vi "Imagen_BN.vi"() -> ()   [LabVIEW 2016]
panel:
  out "Grises":picture
  out "24-bit pixmap":u32[][](array[numeric]) format="%x"
  out "El Poke":picture
  in  "File Path":path
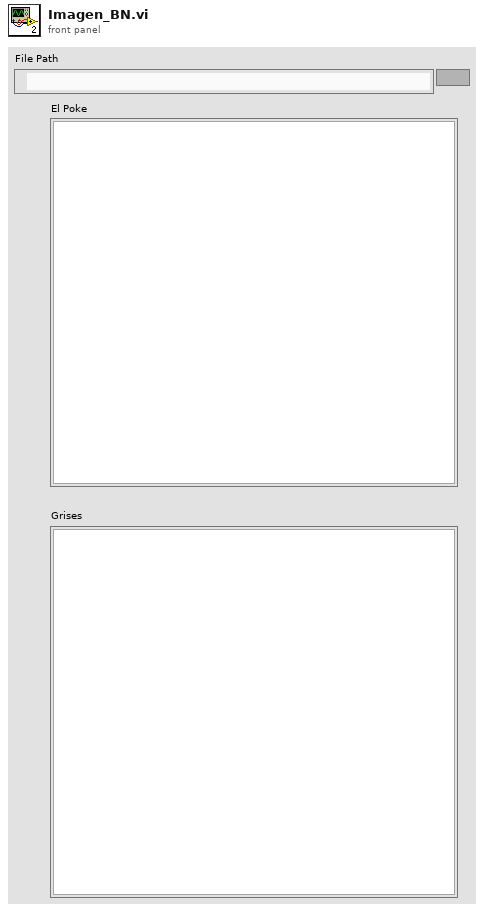
[diagram p1: front panel]
types:
  T1 = typedef "imagedata.ctl" = cluster{"image type":i32, "image depth":i32, "image":u8[], "mask":u8[], "colors":u32[], "Rectangle":cluster{"left":i16, "top":i16, "right":i16, "bottom":i16}}
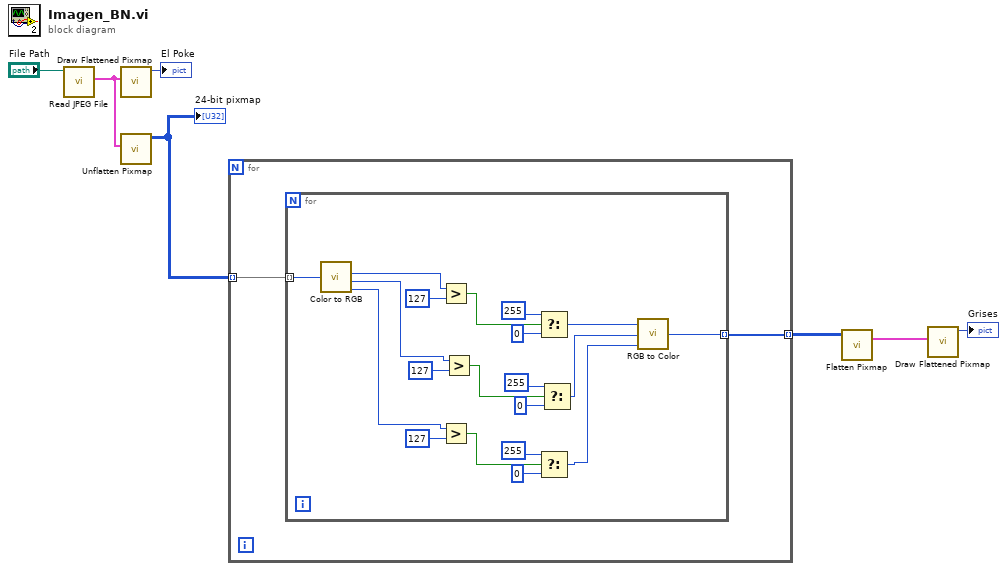
[diagram p0: block diagram]
diagram:
  n1 = call <vilib>:"Read JPEG File.vi"("path to JPEG file"="File Path") -> ("image data"=w5:T1)  [unwired: 8 in, 2 out]
  n2 = call <vilib>:"Draw Flattened Pixmap.vi"("image data"=w5) -> ("new picture"=→"El Poke":picture)  [unwired: 8 in]
  n3 = call <vilib>:"Unflatten Pixmap.vi"("image data"=w5) -> ("24-bit pixmap"=w1:u32[][])  [unwired: 4 in, 6 out]
  "24-bit pixmap" <- w1
  n4 = for {
    tunnel: w1 -> [w9] mode=indexing
    tunnel: [w8] -> w4 mode=indexing
    n5 = for {
      tunnel: w9 -> [w29] mode=indexing
      tunnel: [w10] -> w8 mode=indexing
      n6 = call <vilib>:"Color to RGB.vi"("Color"=w29) -> ("R"=w28:u8, "G"=w18:u8, "B"=w13:u8)  [unwired: 1 out]
      n7 = Greater?(x=w28, y=u8 127) -> (0:w26:bool)
      n8 = Greater?(x=w13, y=u8 127) -> (0:w16:bool)
      n9 = Greater?(x=w18, y=u8 127) -> (0:w21:bool)
      n10 = Select(t=u8 255, s=w26, f=u8 0) -> (s? t:f=w23:u8)
      n11 = Select(t=u8 255, s=w16, f=u8 0) -> (s? t:f=w11:u8)
      n12 = Select(t=u8 255, s=w21, f=u8 0) -> (s? t:f=w12:u8)
      n13 = call <vilib>:"RGB to Color.vi"("B"=w11, "G"=w12, "R"=w23) -> ("Color"=w10:u32)
    }
  }
  n14 = call <vilib>:"Flatten Pixmap.vi"("24-bit pixmap"=w4) -> ("image data"=w2:T1)  [unwired: 10 in]
  n15 = call <vilib>:"Draw Flattened Pixmap.vi"("image data"=w2) -> ("new picture"=→"Grises":picture)  [unwired: 8 in]
